vi "massaj_Simple_EXP.vi"() -> ()   [LabVIEW 2021]
uses:
  PicoMoLV/Global Variablesyes.vi
  C:/Program Files/New Focus/New Focus Picomotor Application/Samples/LabVIEW/Model 8742/LabVIEW 2009/CmdLib.dll
panel:
  in  "SetZero":bool
  out "Output Refnum Out":refnum<vi>
  in  "Set Velocity":dbl(slide)=10.0 min=10.0 max=4000.0 step=10.0 scale=0.0..2500.0
  out "Direction":dbl
  in  "RIGHT":bool caption="CW"
  in  "LEFT":bool
  in  "Decouple":bool
  in  "Stop":bool
  out "error out":errorcluster
  out "In Motion":bool
  out "Status:":string
  out "Current Position:":string
  in  "Go":bool
  in  "Relative Move:":string
  in  "Selected Motor:":string(combo)
  in  "Selected Controller:":string(combo)
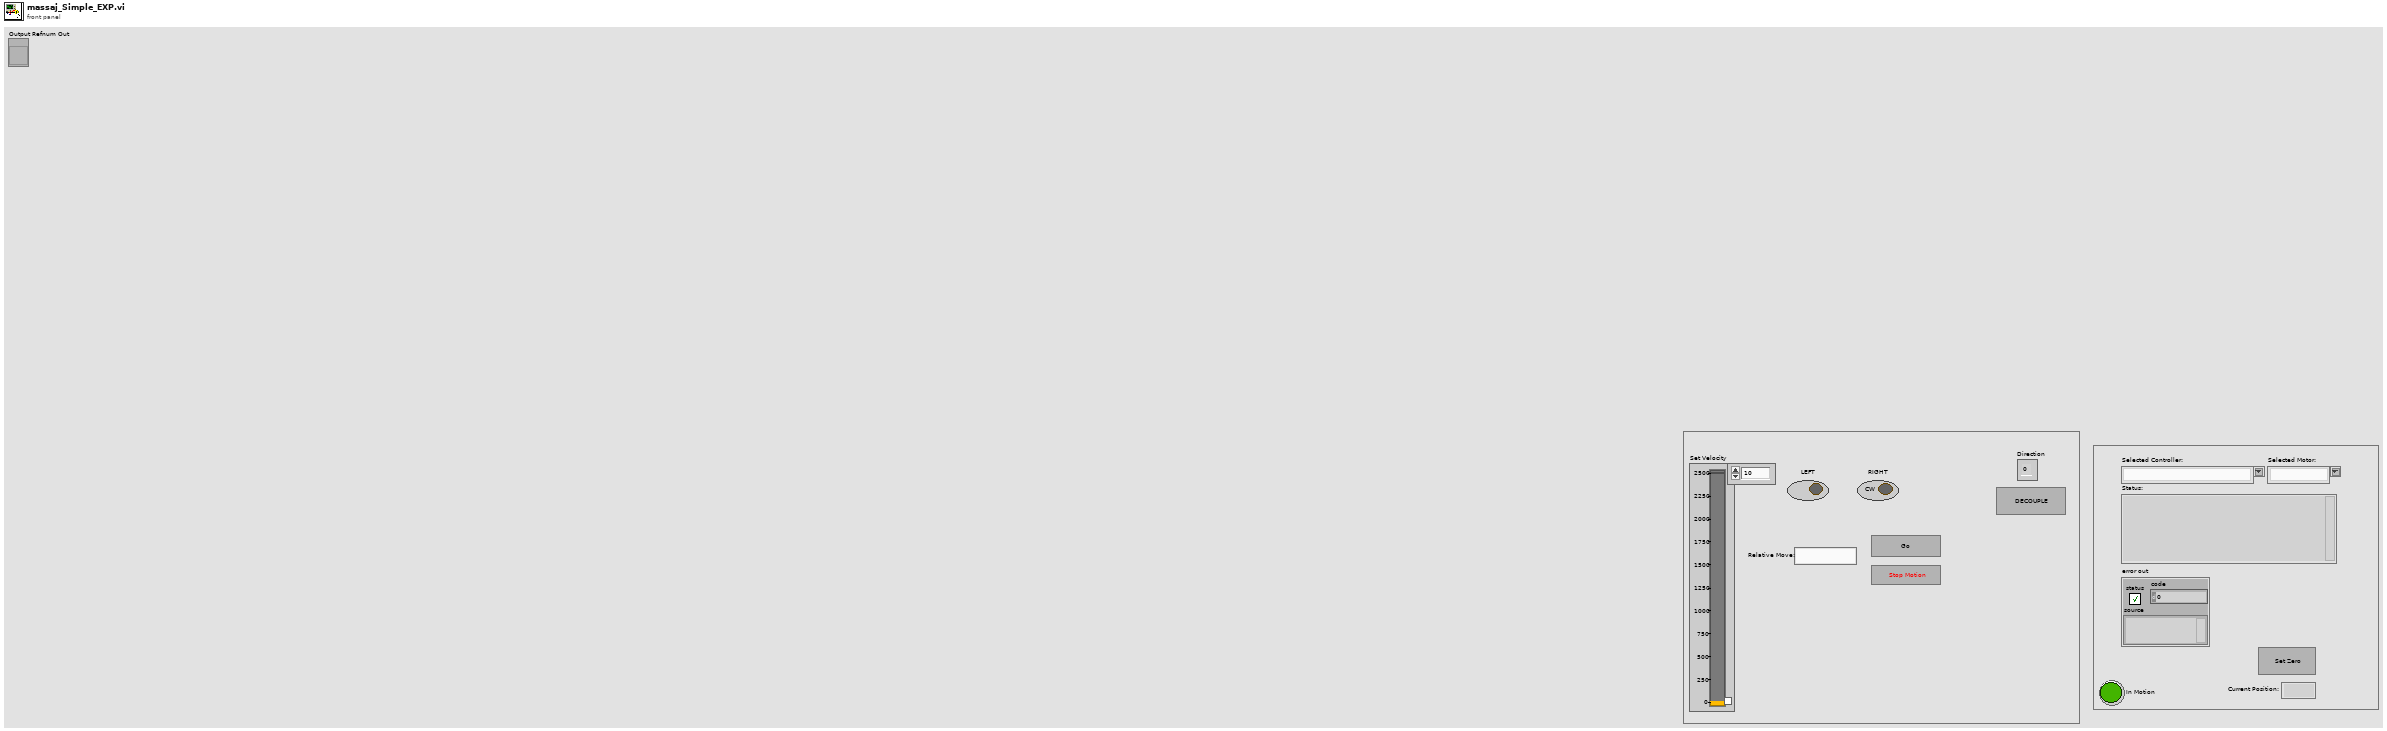
[diagram p1: front panel]
types:
  T1 = cluster{"Selected Controller:":refnum<vi>, "Selected Motor:":refnum<vi>, "Relative Move:":refnum<vi>, "Current Position:":refnum<vi>, "Go":refnum<vi>, "Stop":refnum<vi>}
  T2 = enum8{"Enabled", "Disabled", "Disabled and Grayed Out"}
  T3 = cluster{"DeviceKey":string, "Device Address":i32, "Controller Name":string}[]
  T4 = cluster{"DeviceKey":string, "Device Address":i32, "Controller Name":string}
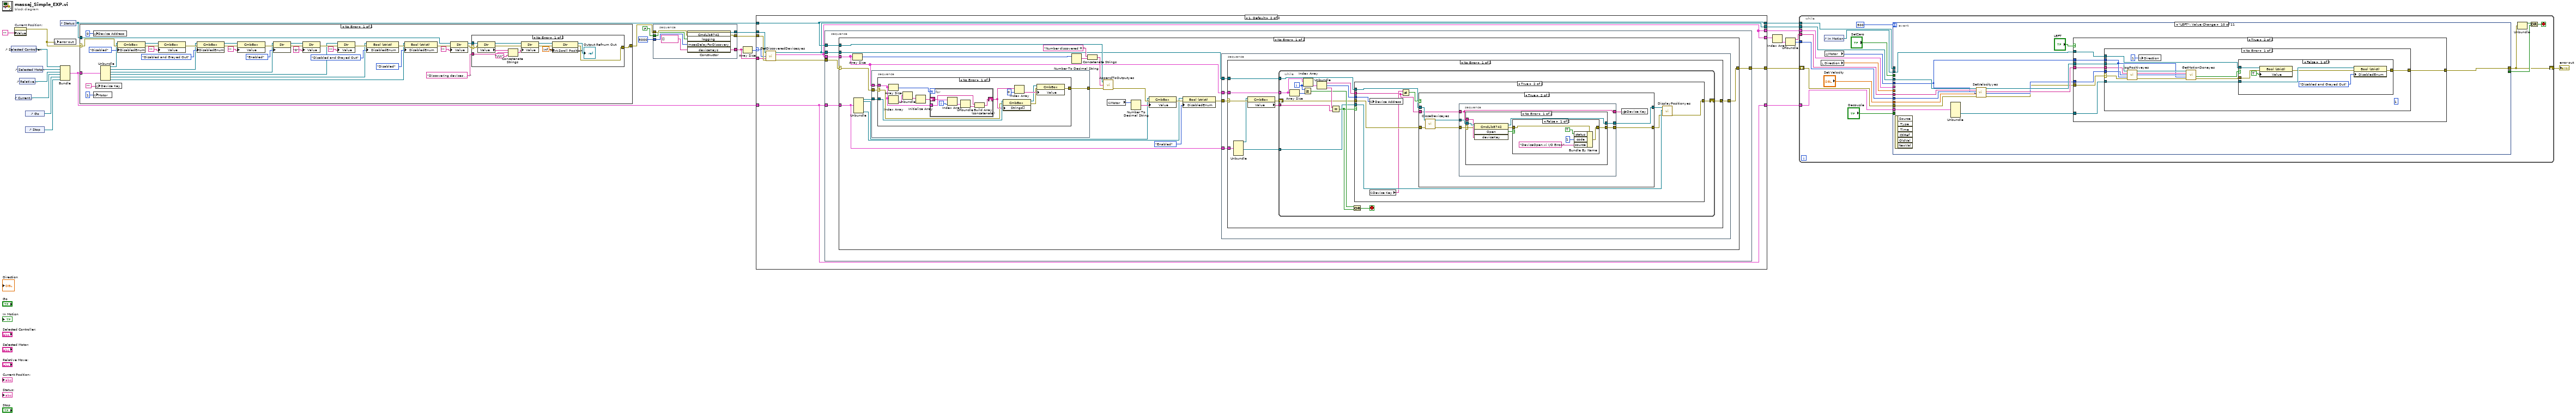
[diagram p0: block diagram]
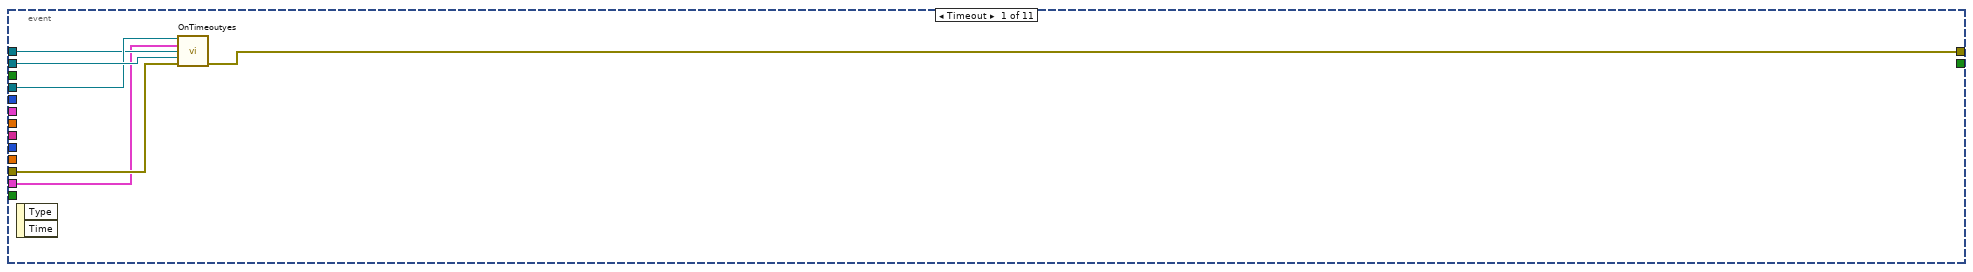
[diagram p4: hidden frame]
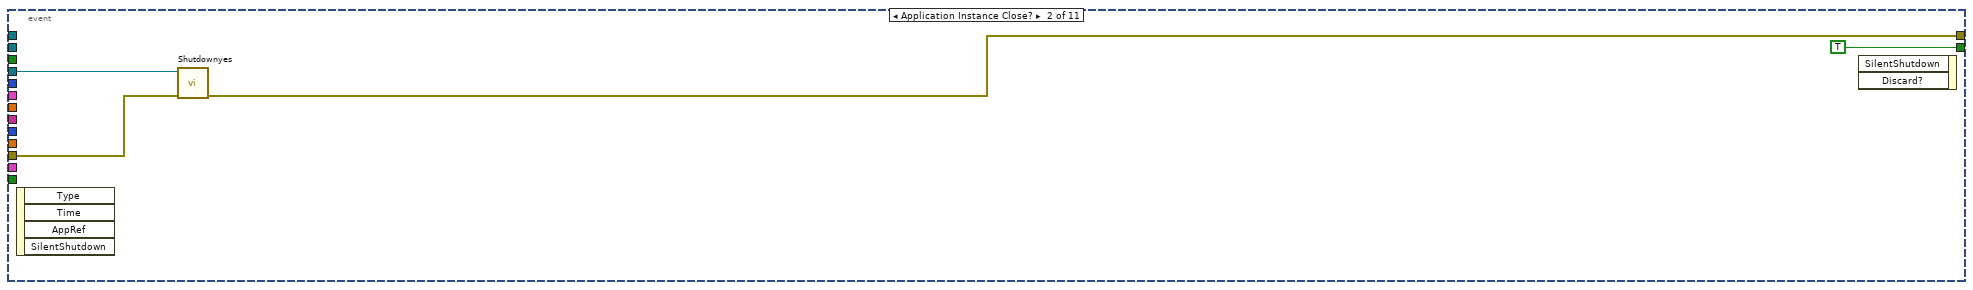
[diagram p5: hidden frame]
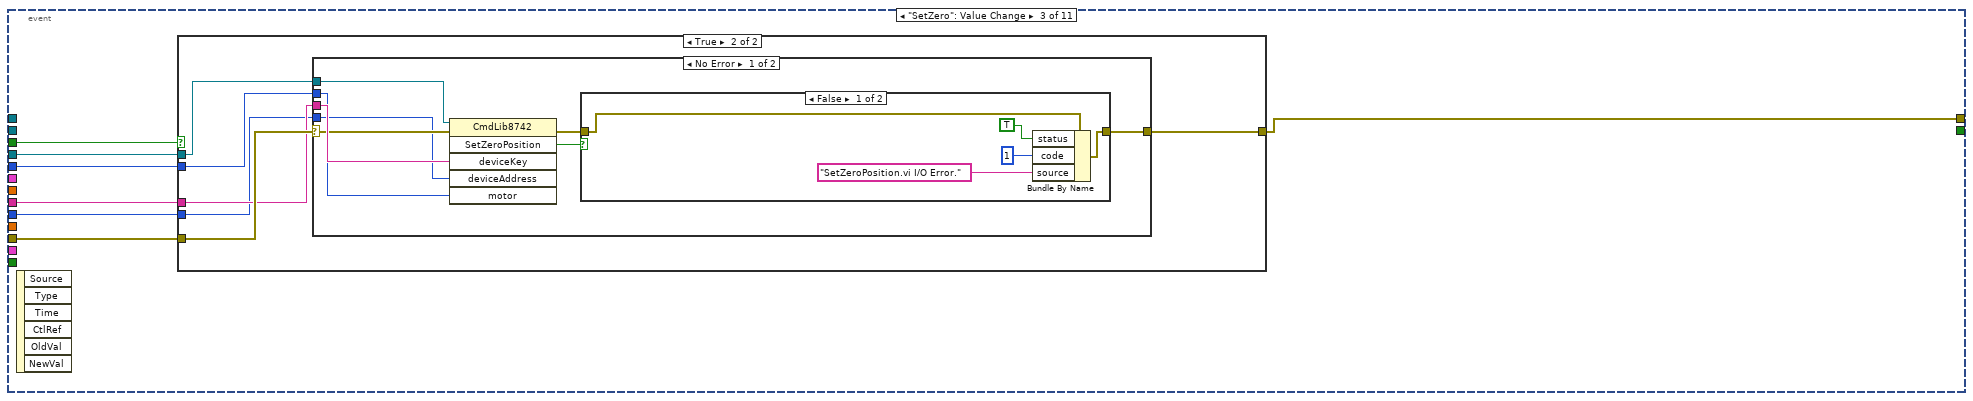
[diagram p6: hidden frame]
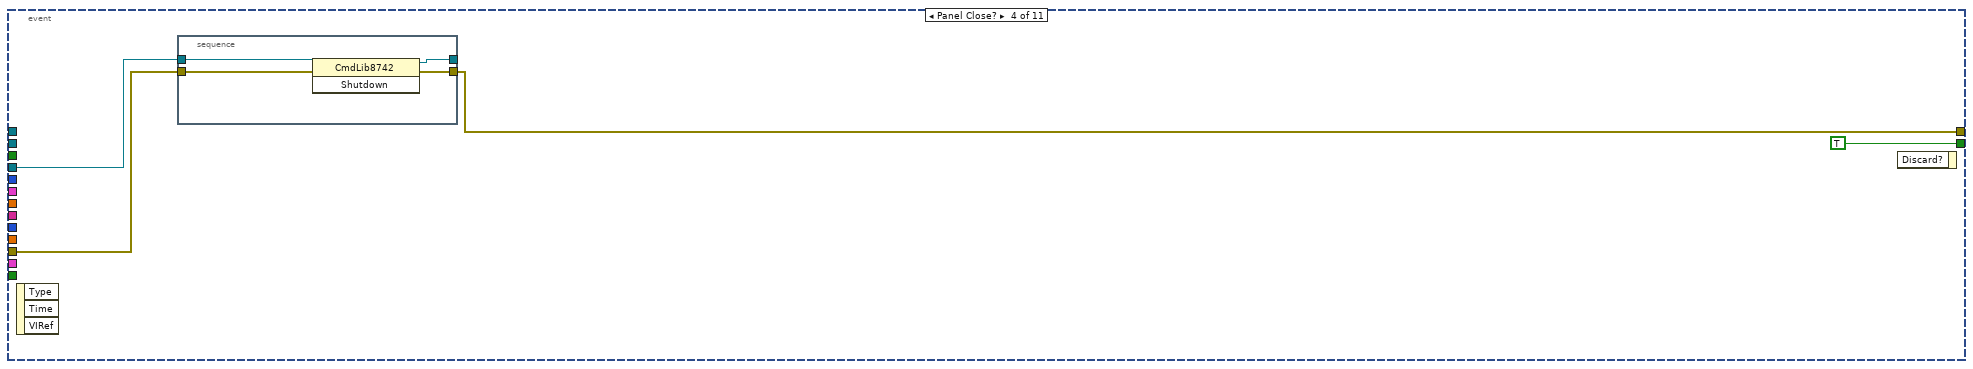
[diagram p10: hidden frame]
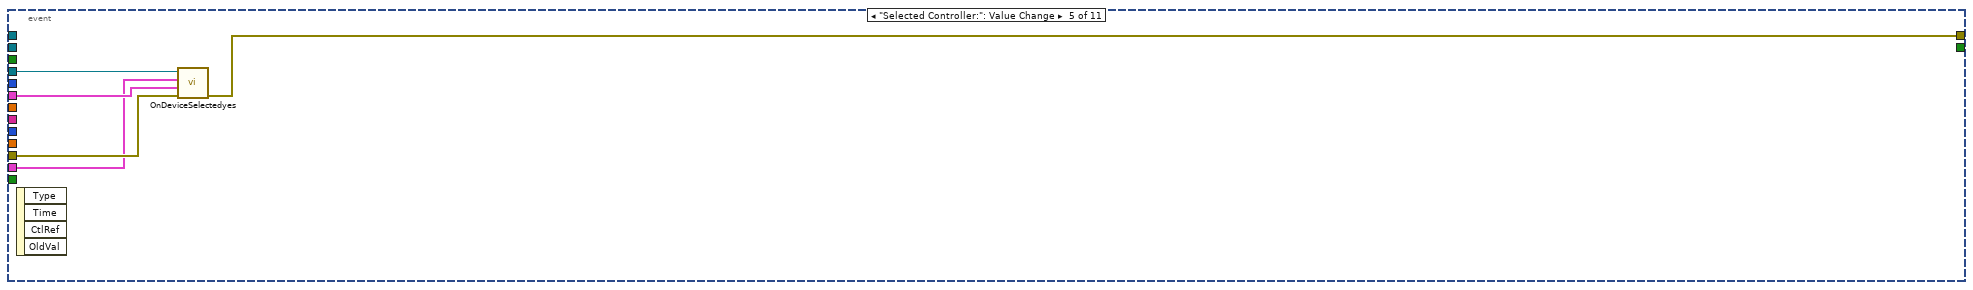
[diagram p11: hidden frame]
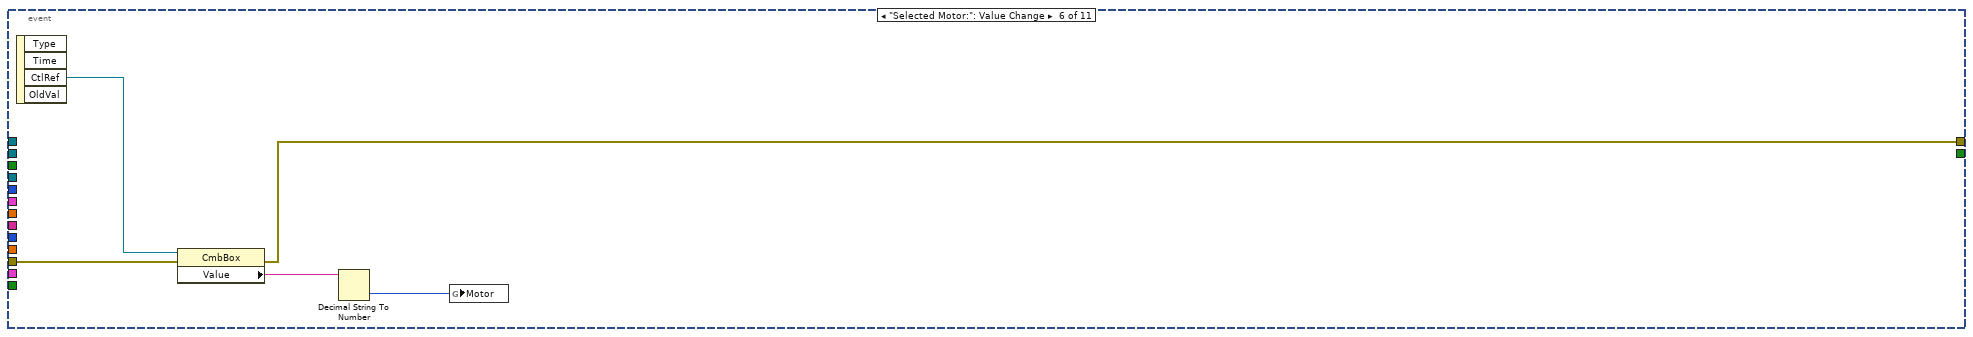
[diagram p12: hidden frame]
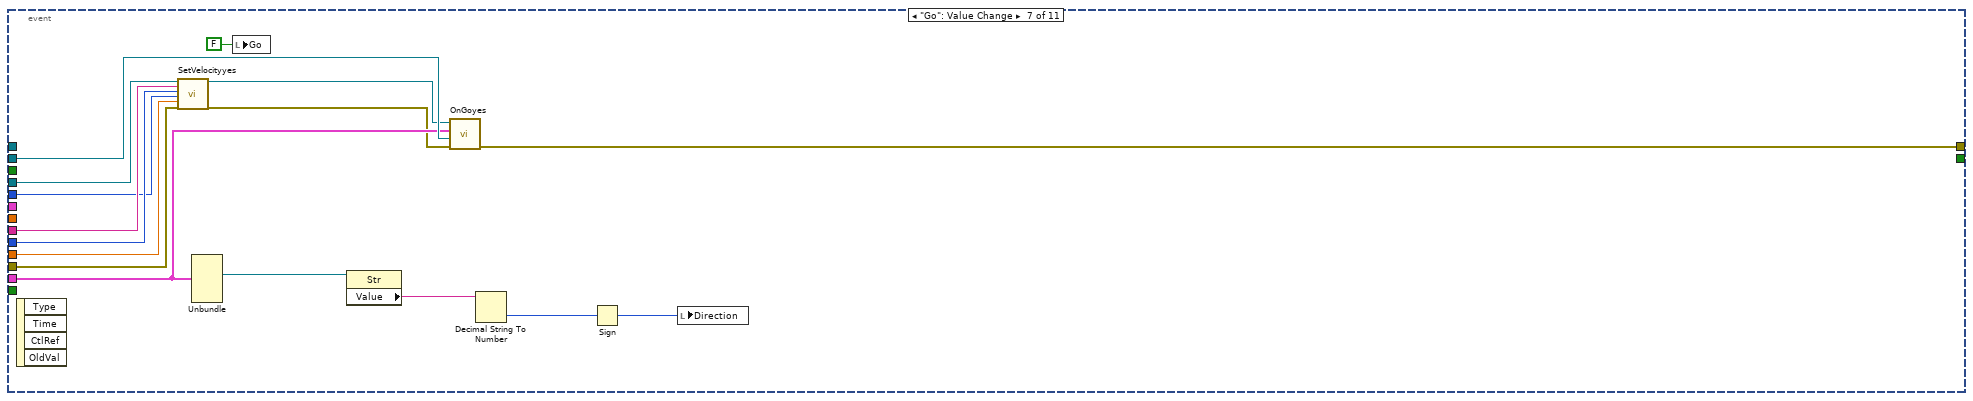
[diagram p13: hidden frame]
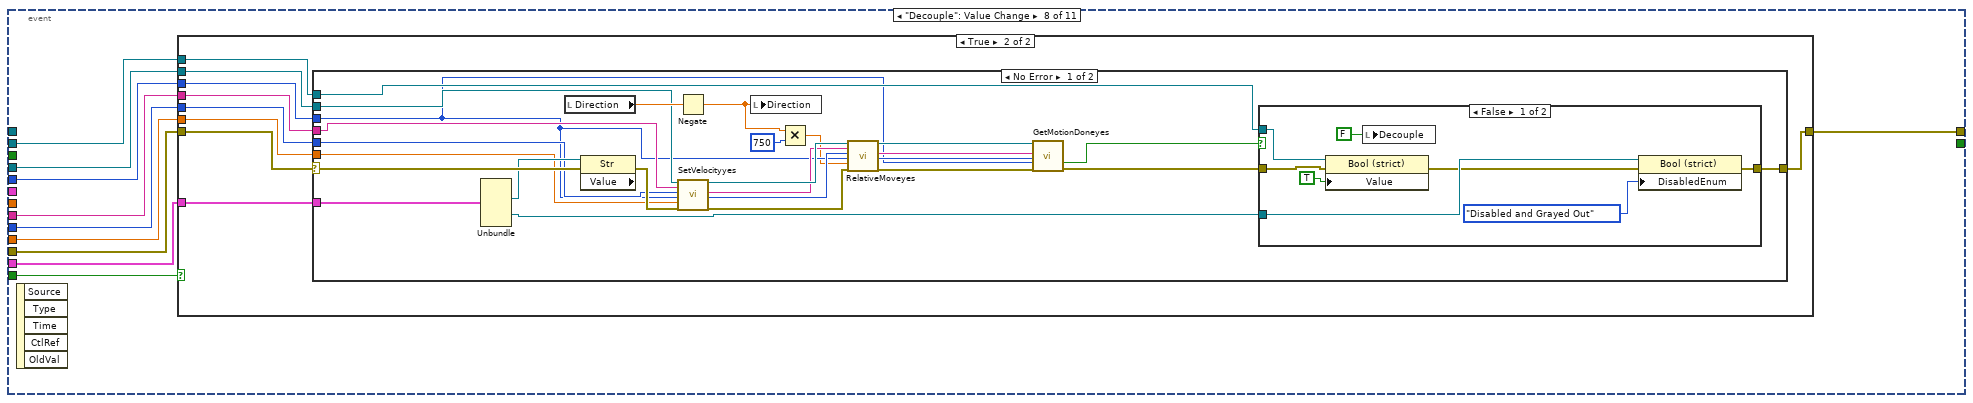
[diagram p14: hidden frame]
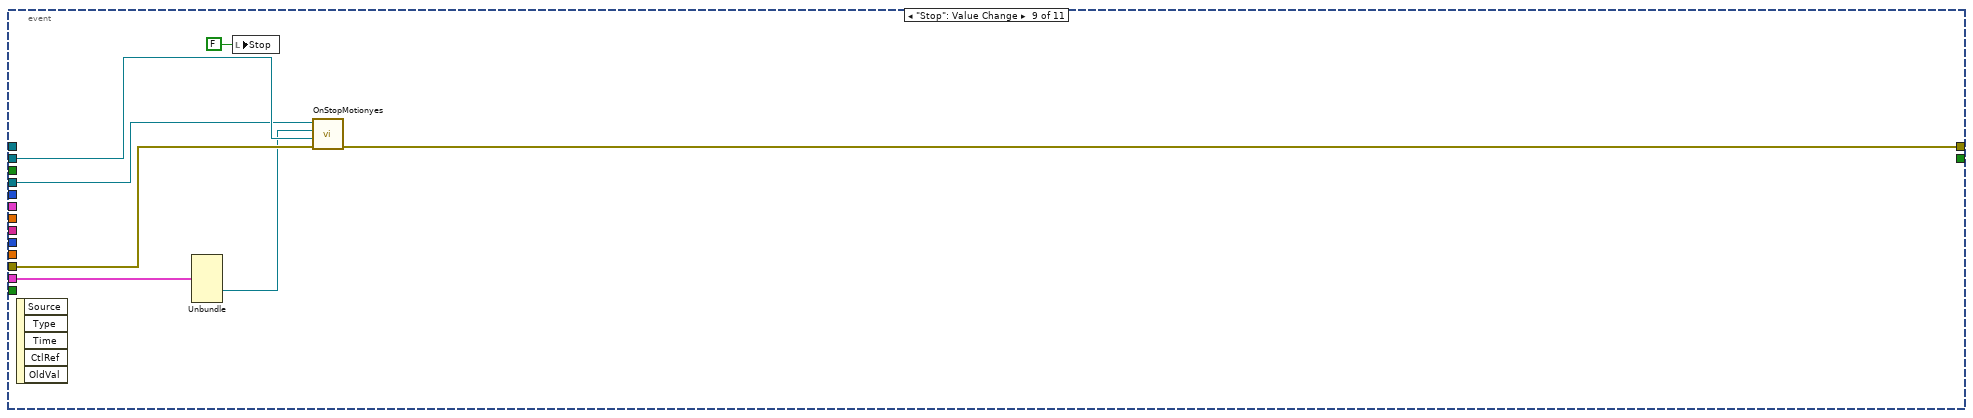
[diagram p18: hidden frame]
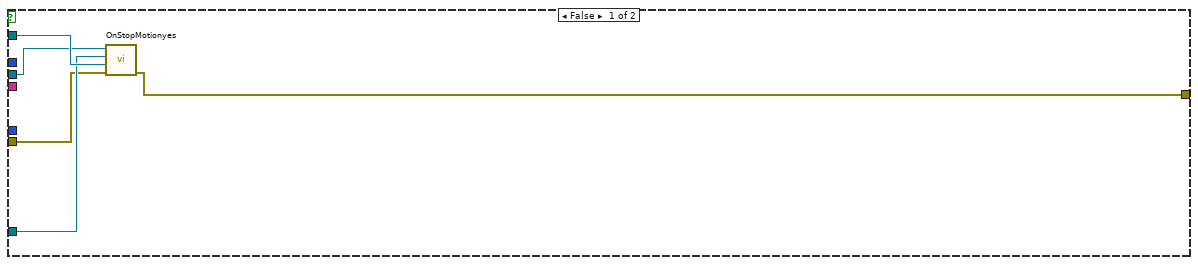
[diagram p19: hidden frame]
diagram:
  n1 = control-ref of="Selected Controller:"() -> (w20:refnum<vi>)
  n2 = property on="Current Position:" class="Str"("Value"="") -> (error out=w10:errorcluster)  [unwired: 2 in, 1 out]
  n3 = control-ref of="Current Position:"() -> (w12:refnum<vi>)
  n4 = control-ref of="Selected Motor:"() -> (w27:refnum<vi>)
  n5 = control-ref of="Relative Move:"() -> (w26:refnum<vi>)
  n6 = control-ref of="Go"() -> (w8:refnum<vi>)
  n7 = control-ref of="Stop"() -> (w9:refnum<vi>)
  n8 = local write "error out"(w10) -> ()
  n9 = Bundle("Selected Controller:"=w20, "Selected Motor:"=w27, "Relative Move:"=w26, "Current Position:"=w12, "Go"=w8, "Stop"=w9) -> (w15:T1)  [unwired: 1 in]
  n10 = control-ref of="Status:"() -> (w19:refnum<vi>)
  n11 = case shown="No Error" w10 {
    selector: w10 -> [w58 w80]
    tunnel: [w28 w80] -> w25
    tunnel: w19 -> [w59 _]
    tunnel: w15 -> [w39 _]
    frame No Error {
      n12 = global write "Global Variablesyes.vi" "Device Address"(0 ("Device Address")) -> ()
      n13 = global write "Global Variablesyes.vi" "Motor"(1 ("Motor")) -> ()
      n14 = global write "Global Variablesyes.vi" "Device Key"("") -> ()
      n15 = Unbundle(w39) -> ("Selected Controller:"=w38:refnum<vi>, "Selected Motor:"=w37:refnum<vi>, "Relative Move:"=w36:refnum<vi>, "Current Position:"=w35:refnum<vi>, "Go"=w34:refnum<vi>, "Stop"=w33:refnum<vi>)
      n16 = property on="Property Node" class="CmbBox"(reference=w38, error in=w58, "DisabledEnum"=T2."Disabled" ("Disabled")) -> (reference out=w57:refnum<vi>, error out=w53:errorcluster)
      n17 = property class="CmbBox"(reference=w57, error in=w53, "Value"="") -> (error out=w52:errorcluster)  [unwired: 1 out]
      n18 = property on="Property Node" class="CmbBox"(reference=w37, error in=w52, "DisabledEnum"=T2."Disabled and Grayed Out" ("Disabled")) -> (reference out=w55:refnum<vi>, error out=w51:errorcluster)
      n19 = property class="CmbBox"(reference=w55, error in=w51, "Value"="") -> (error out=w50:errorcluster)  [unwired: 1 out]
      n20 = property on="Property Node" class="Str"(reference=w36, error in=w50, "DisabledEnum"=T2."Enabled" ("Disabled")) -> (reference out=w46:refnum<vi>, error out=w47:errorcluster)
      n21 = property class="Str"(reference=w46, error in=w47, "Value"="0") -> (error out=w44:errorcluster)  [unwired: 1 out]
      n22 = property on="Property Node" class="Str"(reference=w35, error in=w44, "Value"="") -> (error out=w43:errorcluster)  [unwired: 1 out]
      n23 = property on="Property Node" class="Bool (strict)"(reference=w34, error in=w43, "DisabledEnum"=T2."Disabled and Grayed Out" ("Disabled")) -> (error out=w60:errorcluster)  [unwired: 1 out]
      n24 = property on="Property Node" class="Bool (strict)"(reference=w33, error in=w60, "DisabledEnum"=T2."Disabled" ("Disabled")) -> (error out=w32:errorcluster)  [unwired: 1 out]
      n25 = property class="Str"(reference=w59, error in=w32, "Value"="") -> (reference out=w30:refnum<vi>, error out=w31:errorcluster)
      n26 = case shown="No Error" w31 {
        selector: w31 -> [w73 w79]
        tunnel: [w68 w79] -> w28
        tunnel: w30 -> [w67 _]
        tunnel: "Discovering devices . . ." ("Input String") -> [w66 _]
        frame No Error {
          n27 = property on="Property Node" class="Str"(reference=w67, error in=w73) -> (reference out=w75:refnum<vi>, error out=w74:errorcluster, "Value"=w77:string)
          n28 = Concatenate Strings(w77, w66, "\r\n") -> (w76:string)
          n29 = property class="Str"(reference=w75, error in=w74, "Value"=w76) -> (reference out=w72:refnum<vi>, error out=w71:errorcluster)
          n30 = property class="Str"(reference=w72, error in=w71, "Text.Scroll Position"=inf) -> (reference out=→"Output Refnum Out":refnum<vi>, error out=w68:errorcluster)
        }
        frame Error {
        }
      }
    }
    frame Error {
    }
  }
  n31 = stacked-sequence {
    tunnel: [w81] -> w22
    tunnel: [w86] -> w6
    tunnel: [w82] -> w21
    tunnel: w25 -> [w87]
    tunnel: 5000 ("msecDelayForDiscovery") -> [w84]
    tunnel: FALSE ("logging") -> [w83]
    frame #0 {
      n32 = constructor class="CmdLib8742"(error in=w87, "logging"=w83, "msecDelayForDiscovery"=w84, "deviceKeys"=string[] []) -> (reference out=w82:refnum<k24>, error out=w81:errorcluster, "deviceKeys"=w86:string[])  [unwired: 2 in, 3 out]
    }
  }
  n33 = Array Size(array=w6) -> (size(s)=w23:i32)
  n34 = case shown="1, Default" w23 {
    selector: w23 -> [_ w100]
    tunnel: w19 -> [w89 w97]
    tunnel: w22 -> [w93 w103]
    tunnel: w21 -> [w91 w104]
    tunnel: w6 -> [_ w102]
    tunnel: [w92 w99] -> w18
    tunnel: [w91 w98] -> w17
    tunnel: w15 -> [w90 w96]
    tunnel: [w90 w96] -> w14
    tunnel: [w88 w95] -> w13
    tunnel: [w89 w97] -> w11
    tunnel: [w88 w95] -> w5
    frame 0 {
      w88 = T3 [] ("Device Array")
      n35 = call "AppendToOutputyes.vi"("error in"=w93, "Input String"="No devices were discovered.", "Output Refnum In"=w89) -> ("error out"=w92:errorcluster)  [unwired: 1 in, 1 out]
    }
    frame 1, Default {
      n36 = call "GetDiscoveredDevicesyes.vi"("CmdLib In"=w104, "Master Count"=w100, "DeviceKey List"=w102, "error in"=w103) -> ("CmdLib Out"=w98:refnum<k24>, "Device Array"=w95:T3, "error out"=w101:errorcluster)  [unwired: 9 in]
      n37 = stacked-sequence {
        tunnel: w98 -> [w106]
        tunnel: w97 -> [w108]
        tunnel: w96 -> [w105]
        tunnel: w95 -> [w107]
        tunnel: w101 -> [w110]
        tunnel: [w109] -> w99
        frame #0 {
          n38 = case shown="No Error" w110 {
            selector: w110 -> [w124 w226]
            tunnel: [w126 w226] -> w109
            tunnel: w108 -> [w129 _]
            tunnel: w107 -> [w120 _]
            tunnel: w106 -> [w119 _]
            tunnel: w105 -> [w111 _]
            frame No Error {
              n39 = Array Size(array=w120) -> (size(s)=w125:i32)
              n40 = Unbundle(w111) -> ("Selected Controller:"=w112:refnum<vi>, "Selected Motor:"=w113:refnum<vi>, "Stop"=w114:refnum<vi>)  [unwired: 3 out]
              n41 = stacked-sequence {
                tunnel: [w134] -> w123
                tunnel: w124 -> [w133]
                tunnel: w120 -> [w131]
                tunnel: w112 -> [w132]
                frame #0 {
                  n42 = case shown="No Error" w133 {
                    selector: w133 -> [w135 w154]
                    tunnel: [w136 w154] -> w134
                    tunnel: w132 -> [w145 _]
                    tunnel: w131 -> [w140 _]
                    frame No Error {
                      n43 = Array Size(array=w140) -> (size(s)=w142:i32)
                      n44 = Index Array(array=w140) -> (element=w141:T4)  [unwired: 1 in]
                      n45 = Unbundle(w141) -> ("Controller Name"=w139:string)  [unwired: 2 out]
                      n46 = Initialize Array(w139) -> (w138:string[])  [unwired: 1 in]
                      n47 = for {
                        N: w142 -> [_]
                        tunnel: w140 -> [w153]
                        shift-right: [w149] -> w137
                        shift-left: w138 -> [w150]
                        i -> [w152]
                        n48 = Index Array(array=w153, index=w152) -> (element=w151:T4)
                        n49 = Unbundle(w151) -> ("Controller Name"=w148:string)  [unwired: 2 out]
                        n50 = Build Array (concatenate)(w150, w148) -> (w149:string[])
                      }
                      n51 = property class="CmbBox"(reference=w145, error in=w135, "Strings[]"=w137) -> (reference out=w143:refnum<vi>, error out=w144:errorcluster)
                      n52 = Index Array(array=w137, index=0) -> (element=w147:string)
                      n53 = property class="CmbBox"(reference=w143, error in=w144, "Value"=w147) -> (error out=w136:errorcluster)  [unwired: 1 out]
                    }
                    frame Error {
                    }
                  }
                }
              }
              n54 = Number To Decimal String(number=w125) -> (decimal integer string=w128:string)  [unwired: 1 in]
              n55 = Concatenate Strings("Number discovered = " ("string"), w128) -> (w130:string)
              n56 = call "AppendToOutputyes.vi"("error in"=w123, "Input String"=w130, "Output Refnum In"=w129) -> ("error out"=w118:errorcluster)  [unwired: 1 in, 1 out]
              n57 = global read "Global Variablesyes.vi" "Motor"() -> (w121:i32)
              n58 = Number To Decimal String(number=w121) -> (decimal integer string=w122:string)  [unwired: 1 in]
              n59 = property class="CmbBox"(reference=w113, error in=w118, "Value"=w122) -> (error out=w116:errorcluster)  [unwired: 1 out]
              n60 = property class="Bool (strict)"(reference=w114, error in=w116, "DisabledEnum"=T2."Enabled" ("Disabled")) -> (error out=w115:errorcluster)  [unwired: 1 out]
              n61 = stacked-sequence {
                tunnel: [w158] -> w126
                tunnel: w115 -> [w159]
                tunnel: w120 -> [w157]
                tunnel: w111 -> [w155]
                tunnel: w119 -> [w156]
                frame #0 {
                  n62 = case shown="No Error" w159 {
                    selector: w159 -> [w165 w225]
                    tunnel: [w167 w225] -> w158
                    tunnel: w157 -> [w168 _]
                    tunnel: w156 -> [w164 _]
                    tunnel: w155 -> [w160 _]
                    frame No Error {
                      n63 = Unbundle(w160) -> ("Selected Controller:"=w162:refnum<vi>, "Current Position:"=w161:refnum<vi>)  [unwired: 4 out]
                      n64 = property class="CmbBox"(reference=w162, error in=w165) -> (error out=w163:errorcluster, "Value"=w166:string)  [unwired: 1 out]
                      n65 = while {
                        tunnel: w168 -> [w182]
                        tunnel: w166 -> [w169]
                        tunnel: w161 -> [w171]
                        shift-right: [w173] -> w167
                        shift-left: w163 -> [w172]
                        tunnel: w164 -> [w170]
                        i -> [w181]
                        stop <- w176 stop-if-true
                        n66 = Array Size(array=w182) -> (size(s)=w183:i32)
                        n67 = Greater Or Equal?(x=w181, y=w183) -> (x >= y?=w178:bool)
                        n68 = Index Array(array=w182, index=w181) -> (element=w180:T4)
                        n69 = Unbundle(w180) -> ("DeviceKey"=w175:string, "Device Address"=w174:i32, "Controller Name"=w179:string)
                        n70 = Equal?(x=w179, y=w169) -> (x = y?=w177:bool)
                        n71 = Or(x=w178, y=w177) -> (x .or. y?=w176:bool)
                        n72 = case shown="True" w177 {
                          tunnel: w175 -> [_ w190]
                          tunnel: w174 -> [_ w185]
                          tunnel: [w184 w194] -> w173
                          tunnel: w172 -> [w184 w192]
                          tunnel: w171 -> [_ w193]
                          tunnel: w170 -> [_ w188]
                          frame False {
                          }
                          frame True {
                            n73 = global write "Global Variablesyes.vi" "Device Address"(w185) -> ()
                            n74 = global read "Global Variablesyes.vi" "Device Key"() -> (w191:string)
                            n75 = Not Equal?(x=w191, y=w190) -> (x != y?=w189:bool)
                            n76 = case shown="True" w189 {
                              tunnel: [w196 w198] -> w186
                              tunnel: w188 -> [w195 w204]
                              tunnel: w192 -> [w196 w202]
                              tunnel: w190 -> [_ w200]
                              tunnel: [w195 w197] -> w187
                              frame False {
                              }
                              frame True {
                                n77 = call "CloseDeviceyes.vi"("error in"=w202, "CmdLib In"=w204) -> ("error out"=w203:errorcluster, "CmdLib Out"=w201:refnum<k24>)  [unwired: 8 in]
                                n78 = stacked-sequence {
                                tunnel: [w209] -> w198
                                tunnel: [w207] -> w199
                                tunnel: [w206] -> w197
                                tunnel: w203 -> [w208]
                                tunnel: w200 -> [w207]
                                tunnel: w201 -> [w205]
                                frame #0 {
                                n79 = case shown="No Error" w208 {
                                selector: w208 -> [w213 w224]
                                tunnel: w205 -> [w216 w223]
                                tunnel: [w215 w223] -> w206
                                tunnel: w207 -> [w214 _]
                                tunnel: [w210 w224] -> w209
                                frame No Error {
                                n80 = invoke class="CmdLib8742" method="Open"(reference=w216, error in=w213, "deviceKey"=w214) -> (reference out=w215:refnum<k24>, error out=w211:errorcluster, "Open"=w212:bool)  [unwired: 1 in, 1 out]
                                n81 = case shown="False" w212 {
                                tunnel: w211 -> [w219 w222]
                                tunnel: [w218 w222] -> w210
                                frame False {
                                n82 = Bundle By Name(cluster=w219, "status"=TRUE, "code"=1, "source"="DeviceOpen.vi I/O Error.") -> (w218:errorcluster)
                                }
                                frame True {
                                }
                                }
                                }
                                frame Error {
                                }
                                }
                                }
                                }
                                n83 = global write "Global Variablesyes.vi" "Device Key"(w199) -> ()
                              }
                            }
                            n84 = call "DisplayPositionyes.vi"("error in"=w186, "Current Position:"=w193, "CmdLib In"=w187) -> ("error out"=w194:errorcluster)  [unwired: 7 in, 1 out]
                          }
                        }
                      }
                    }
                    frame Error {
                    }
                  }
                }
              }
            }
            frame Error {
            }
          }
        }
      }
    }
  }
  n85 = Index Array(array=w5) -> (element=w4:T4)  [unwired: 1 in]
  n86 = Unbundle(w4) -> ("DeviceKey"=w3:string, "Device Address"=w1:i32)  [unwired: 1 out]
  n87 = while {
    tunnel: w17 -> [w243]
    tunnel: w14 -> [w242]
    tunnel: w13 -> [w241]
    shift-right: [w235] -> w7
    shift-left: w18 -> [w244]
    tunnel: w11 -> [w239]
    tunnel: w3 -> [w229]
    tunnel: w1 -> [w227]
    stop <- w234 stop-if-true
    n88 = local read "Direction"() -> (w232:dbl)
    n89 = control-ref of="In Motion"() -> (w236:refnum<vi>)
    n90 = global read "Global Variablesyes.vi" "Motor"() -> (w231:i32)
    n91 = event shown="[9] \"LEFT\": Value Change" {
      selector: _ -> [_ _ _ _ _ _ _ _ _ _ _]
      dyn-events: _ -> [_ _ _ _ _ _ _ _ _ _ _]
      timeout: 500 -> [_ _ _ _ _ _ _ _ _ _ _]
      tunnel: w244 -> [w250 w254 w260 w286 w296 w299 w303 w324 w378 w394 w439]
      tunnel: w243 -> [w247 w253 w255 w287 w293 _ w309 w326 w374 w392 w440]
      tunnel: [_ TRUE _ TRUE _ _ _ _ _ _ _] -> w237
      tunnel: [w249 w251 w256 w284 w295 w298 w315 w323 w377 w389 _] -> w235
      tunnel: w242 -> [w245 _ _ _ w292 _ w314 w327 w376 w390 w441]
      tunnel: w241 -> [_ _ _ _ w294 _ _ _ _ _ _]
      tunnel: w239 -> [w246 _ _ _ _ _ _ _ _ _ _]
      tunnel: w236 -> [w248 _ _ _ _ _ w317 w325 w379 w395 w438]
      tunnel: "Decouple" -> [_ _ _ _ _ _ _ w318 _ _ _]
      tunnel: w232 -> [_ _ _ _ _ _ _ _ _ _ _]
      tunnel: w231 -> [_ _ w259 _ _ _ w305 w320 _ w381 w434]
      tunnel: w229 -> [_ _ w258 _ _ _ w307 w322 _ w388 w435]
      tunnel: w227 -> [_ _ w257 _ _ _ w306 w321 _ w387 w436]
      tunnel: "Set Velocity" -> [_ _ _ _ _ _ w304 w319 _ w382 w433]
      tunnel: "SetZero" -> [_ _ w261 _ _ _ _ _ _ _ _]
      event Timeout {
        n92 = event-data() -> ()  [unwired: 1 in, 2 out]
        n93 = call "OnTimeoutyes.vi"("CmdLib In"=w247, "UI"=w245, "Status:"=w246, "In Motion"=w248, "error in"=w250) -> ("error out"=w249:errorcluster)  [unwired: 10 in]
      }
      event Application Instance Close? {
        n94 = event-data() -> ()  [unwired: 1 in, 4 out]
        n95 = call "Shutdownyes.vi"("error in (no error)"=w254, "CmdLib In"=w253) -> ("error out"=w251:errorcluster)  [unwired: 4 in, 1 out]
        n96 = event-data() -> ()  [unwired: 3 in, 1 out]
      }
      event "SetZero": Value Change {
        n97 = event-data() -> ()  [unwired: 1 in, 6 out]
        n98 = case shown="True" w261 {
          tunnel: w260 -> [w262 w268]
          tunnel: w259 -> [_ w267]
          tunnel: w258 -> [_ w266]
          tunnel: w257 -> [_ w265]
          tunnel: [w262 w264] -> w256
          tunnel: w255 -> [_ w263]
          frame False {
          }
          frame True {
            n99 = case shown="No Error" w268 {
              selector: w268 -> [w274 w283]
              tunnel: w263 -> [w276 _]
              tunnel: w267 -> [w270 _]
              tunnel: w266 -> [w275 _]
              tunnel: [w271 w283] -> w264
              tunnel: w265 -> [w269 _]
              frame No Error {
                n100 = invoke class="CmdLib8742" method="SetZeroPosition"(reference=w276, error in=w274, "deviceKey"=w275, "deviceAddress"=w269, "motor"=w270) -> (error out=w272:errorcluster, "SetZeroPosition"=w273:bool)  [unwired: 1 in, 4 out]
                n101 = case shown="False" w273 {
                  tunnel: w272 -> [w281 w282]
                  tunnel: [w280 w282] -> w271
                  frame False {
                    n102 = Bundle By Name(cluster=w281, "status"=TRUE, "code"=1, "source"="SetZeroPosition.vi I/O Error.") -> (w280:errorcluster)
                  }
                  frame True {
                  }
                }
              }
              frame Error {
              }
            }
          }
        }
      }
      event Panel Close? {
        n103 = event-data() -> ()  [unwired: 1 in, 3 out]
        n104 = stacked-sequence {
          tunnel: [w291] -> w284
          tunnel: [w288] -> _
          tunnel: w286 -> [w290]
          tunnel: w287 -> [w289]
          frame #0 {
            n105 = invoke class="CmdLib8742" method="Shutdown"(reference=w289, error in=w290) -> (reference out=w288:refnum<k24>, error out=w291:errorcluster)  [unwired: 1 in, 1 out]
          }
        }
        n106 = event-data() -> ()  [unwired: 2 in, 1 out]
      }
      event "Selected Controller:": Value Change {
        n107 = event-data() -> ()  [unwired: 1 in, 4 out]
        n108 = call "OnDeviceSelectedyes.vi"("error in"=w296, "Device Array"=w294, "UI"=w292, "CmdLib In"=w293) -> ("error out"=w295:errorcluster)  [unwired: 7 in]
      }
      event "Selected Motor:": Value Change {
        n109 = event-data() -> ("CtlRef"=w297:refnum<vi>)  [unwired: 1 in, 3 out]
        n110 = property class="CmbBox"(reference=w297, error in=w299) -> (error out=w298:errorcluster, "Value"=w301:string)  [unwired: 1 out]
        n111 = Decimal String To Number(string=w301) -> (number=w300:i32)  [unwired: 2 in, 1 out]
        n112 = global write "Global Variablesyes.vi" "Motor"(w300) -> ()
      }
      event "Go": Value Change {
        n113 = event-data() -> ()  [unwired: 1 in, 4 out]
        n114 = call "SetVelocityyes.vi"("CmdLib In"=w309, "DeviceKey In"=w307, "Device Address In"=w306, "Motor"=w305, "Steps Per Sec"=w304, "error in (no error)"=w303) -> ("CmdLib Out"=w308:refnum<k24>, "error out"=w302:errorcluster)  [unwired: 10 in, 2 out]
        n115 = Unbundle(w314) -> ("Relative Move:"=w312:refnum<vi>)  [unwired: 5 out]
        n116 = local write "Go"(FALSE ("Go")) -> ()
        n117 = property class="Str"(reference=w312) -> ("Value"=w313:string)  [unwired: 1 in, 2 out]
        n118 = call "OnGoyes.vi"("error in"=w302, "In Motion"=w317, "UI"=w314, "CmdLib Out"=w308) -> ("error out"=w315:errorcluster)  [unwired: 7 in]
        n119 = Decimal String To Number(string=w313) -> (number=w311:i32)  [unwired: 2 in, 1 out]
        n120 = Sign(1:w311) -> (0:w310:i32)
        n121 = local write "Direction"(w310) -> ()
      }
      event "Decouple": Value Change {
        n122 = event-data() -> ()  [unwired: 1 in, 5 out]
        n123 = case shown="True" w318 {
          tunnel: w327 -> [_ w337]
          tunnel: w326 -> [_ w336]
          tunnel: w325 -> [_ w335]
          tunnel: w324 -> [w328 w334]
          tunnel: [w328 w333] -> w323
          tunnel: w322 -> [_ w332]
          tunnel: w321 -> [_ w331]
          tunnel: w320 -> [_ w330]
          tunnel: w319 -> [_ w329]
          frame False {
          }
          frame True {
            n124 = case shown="No Error" w334 {
              selector: w334 -> [w360 w373]
              tunnel: [w361 w373] -> w333
              tunnel: w337 -> [w357 _]
              tunnel: w336 -> [w351 _]
              tunnel: w335 -> [w356 _]
              tunnel: w332 -> [w348 _]
              tunnel: w331 -> [w347 _]
              tunnel: w330 -> [w341 _]
              tunnel: w329 -> [w342 _]
              frame No Error {
                n125 = Unbundle(w357) -> ("Relative Move:"=w358:refnum<vi>, "Go"=w359:refnum<vi>)  [unwired: 4 out]
                n126 = local read "Direction"() -> (w355:dbl)
                n127 = property class="Str" props=["Value"](reference=w358, error in=w360) -> (error out=w354:errorcluster)  [unwired: 2 out]
                n128 = Negate(x=w355) -> (-x=w339:dbl)
                n129 = call "SetVelocityyes.vi"("CmdLib In"=w351, "DeviceKey In"=w348, "Device Address In"=w347, "Motor"=w341, "Steps Per Sec"=w342, "error in (no error)"=w354) -> ("CmdLib Out"=w350:refnum<k24>, "DeviceKey Out"=w346:string, "Device Address Out"=w344:i32, "error out"=w353:errorcluster)  [unwired: 10 in]
                n130 = local write "Direction"(w339) -> ()
                n131 = Multiply(x=w339, y=750) -> (x*y=w338:dbl)
                n132 = call "RelativeMoveyes.vi"("CmdLib In"=w350, "DeviceKey In"=w346, "Device Address In"=w344, "Motor"=w341, "Relative Steps"=w338, "error in (no error)"=w353) -> ("CmdLib Out"=w349:refnum<k24>, "DeviceKey Out"=w345:string, "Device Address Out"=w343:i32, "error out"=w352:errorcluster)  [unwired: 10 in]
                n133 = call "GetMotionDoneyes.vi"("CmdLib In"=w349, "DeviceKey In"=w345, "Device Address In"=w343, "Motor"=w341, "error in (no error)"=w352) -> ("Is Motion Done"=w363:bool, "error out"=w362:errorcluster)  [unwired: 6 in, 3 out]
                n134 = case shown="False" w363 {
                  tunnel: [w365 w372] -> w361
                  tunnel: w359 -> [w370 _]
                  tunnel: w362 -> [w367 w372]
                  tunnel: w356 -> [w369 _]
                  frame False {
                    n135 = property class="Bool (strict)"(reference=w369, error in=w367, "Value"=TRUE) -> (error out=w366:errorcluster)  [unwired: 1 out]
                    n136 = local write "Decouple"(FALSE) -> ()
                    n137 = property class="Bool (strict)"(reference=w370, error in=w366, "DisabledEnum"=T2."Disabled and Grayed Out" ("Disabled")) -> (error out=w365:errorcluster)  [unwired: 1 out]
                  }
                  frame True {
                  }
                }
              }
              frame Error {
              }
            }
          }
        }
      }
      event "Stop": Value Change {
        n138 = event-data() -> ()  [unwired: 1 in, 5 out]
        n139 = Unbundle(w376) -> ("Go"=w375:refnum<vi>)  [unwired: 5 out]
        n140 = local write "Stop"(FALSE) -> ()
        n141 = call "OnStopMotionyes.vi"("error in"=w378, "In Motion"=w379, "Go"=w375, "CmdLib In"=w374) -> ("error out"=w377:errorcluster)  [unwired: 7 in]
      }
      event "LEFT": Value Change {
        n142 = event-data() -> ()  [unwired: 1 in, 6 out]
        n143 = Unbundle(w390) -> ("Go"=w391:refnum<vi>)  [unwired: 5 out]
        n144 = call "SetVelocityyes.vi"("CmdLib In"=w392, "DeviceKey In"=w388, "Device Address In"=w387, "Motor"=w381, "Steps Per Sec"=w382, "error in (no error)"=w394) -> ("CmdLib Out"=w386:refnum<k24>, "DeviceKey Out"=w385:string, "Device Address Out"=w384:i32, "error out"=w383:errorcluster)  [unwired: 10 in]
        n145 = case shown="True" "LEFT" {
          tunnel: w395 -> [w400 w408]
          tunnel: [w399 w407] -> w389
          tunnel: w391 -> [w398 w406]
          tunnel: w381 -> [_ w405]
          tunnel: w386 -> [w396 w404]
          tunnel: w385 -> [_ w403]
          tunnel: w384 -> [_ w402]
          tunnel: w383 -> [w397 w401]
          frame False {
            n146 = call "OnStopMotionyes.vi"("error in"=w397, "In Motion"=w400, "Go"=w398, "CmdLib In"=w396) -> ("error out"=w399:errorcluster)  [unwired: 7 in]
          }
          frame True {
            n147 = case shown="No Error" w401 {
              selector: w401 -> [w409 w432]
              tunnel: [w421 w432] -> w407
              tunnel: w408 -> [w420 _]
              tunnel: w406 -> [w419 _]
              tunnel: w405 -> [w413 _]
              tunnel: w404 -> [w412 _]
              tunnel: w403 -> [w411 _]
              tunnel: w402 -> [w410 _]
              frame No Error {
                (unwired) 1
                n148 = call "JogPositiveyes.vi"("CmdLib In"=w412, "DeviceKey In"=w411, "Device Address In"=w410, "Motor"=w413, "error in (no error)"=w409) -> ("CmdLib Out"=w417:refnum<k24>, "DeviceKey Out"=w416:string, "Device Address Out"=w415:i32, "error out"=w414:errorcluster)  [unwired: 7 in]
                n149 = local write "Direction"(1) -> ()
                n150 = call "GetMotionDoneyes.vi"("CmdLib In"=w417, "DeviceKey In"=w416, "Device Address In"=w415, "Motor"=w413, "error in (no error)"=w414) -> ("Is Motion Done"=w423:bool, "error out"=w422:errorcluster)  [unwired: 6 in, 3 out]
                n151 = case shown="False" w423 {
                  tunnel: [w424 w431] -> w421
                  tunnel: w419 -> [w429 _]
                  tunnel: w422 -> [w426 w431]
                  tunnel: w420 -> [w428 _]
                  frame False {
                    n152 = property class="Bool (strict)"(reference=w428, error in=w426, "Value"=TRUE) -> (error out=w425:errorcluster)  [unwired: 1 out]
                    n153 = property class="Bool (strict)"(reference=w429, error in=w425, "DisabledEnum"=T2."Disabled and Grayed Out" ("Disabled")) -> (error out=w424:errorcluster)  [unwired: 1 out]
                  }
                  frame True {
                  }
                }
              }
              frame Error {
              }
            }
          }
        }
      }
      event "RIGHT": Value Change {
        n154 = event-data() -> ()  [unwired: 1 in, 6 out]
        n155 = Unbundle(w441) -> ("Go"=w442:refnum<vi>)  [unwired: 5 out]
        n156 = case shown="True" "RIGHT" {
          tunnel: w440 -> [w447 w456]
          tunnel: w438 -> [w446 w455]
          tunnel: w439 -> [w445 w454]
          tunnel: [w444 w453] -> _
          tunnel: w442 -> [w443 w452]
          tunnel: w436 -> [_ w451]
          tunnel: w435 -> [_ w450]
          tunnel: w434 -> [_ w449]
          tunnel: w433 -> [_ w448]
          frame False {
            n157 = call "OnStopMotionyes.vi"("error in"=w445, "In Motion"=w446, "Go"=w443, "CmdLib In"=w447) -> ("error out"=w444:errorcluster)  [unwired: 7 in]
          }
          frame True {
            n158 = case shown="No Error" w454 {
              selector: w454 -> [w466 w482]
              tunnel: [w467 w482] -> w453
              tunnel: w456 -> [w465 _]
              tunnel: w455 -> [w464 _]
              tunnel: w452 -> [w463 _]
              tunnel: w451 -> [w460 _]
              tunnel: w450 -> [w459 _]
              tunnel: w449 -> [w458 _]
              tunnel: w448 -> [w457 _]
              frame No Error {
                n159 = call "Couplingvi.vi"("Motor"=w458, "Step per Sec"=w457, "Device Key"=w459, "error in (no error)"=w466, "LEFT/RIGHT COUPLE"=FALSE, "Device Address"=w460, ".NET Refnum in"=w465) -> ("error out"=w468:errorcluster, "Device Address Out"=w472:i32, "DeviceKey Out"=w471:string, ".NET Refnum out"=w470:refnum<k24>, "Direction"=w461:i32)
                n160 = call "GetMotionDoneyes.vi"("CmdLib In"=w470, "DeviceKey In"=w471, "Device Address In"=w472, "Motor"=w458, "error in (no error)"=w468) -> ("Is Motion Done"=w473:bool, "error out"=w469:errorcluster)  [unwired: 6 in, 3 out]
                n161 = local write "Direction"(w461) -> ()
                n162 = case shown="False" w473 {
                  tunnel: [w474 w481] -> w467
                  tunnel: w463 -> [w479 _]
                  tunnel: w469 -> [w476 w481]
                  tunnel: w464 -> [w478 _]
                  frame False {
                    n163 = property class="Bool (strict)"(reference=w478, error in=w476, "Value"=TRUE) -> (error out=w475:errorcluster)  [unwired: 1 out]
                    n164 = property class="Bool (strict)"(reference=w479, error in=w475, "DisabledEnum"=T2."Disabled and Grayed Out" ("Disabled")) -> (error out=w474:errorcluster)  [unwired: 1 out]
                  }
                  frame True {
                  }
                }
              }
              frame Error {
              }
            }
          }
        }
      }
    }
    n165 = Unbundle(w235) -> ("status"=w238:bool)  [unwired: 2 out]
    n166 = Or(x=w238, y=w237) -> (x .or. y?=w234:bool)
  }
  "error out" <- w7
